vi "4.7.vi"() -> ()   [LabVIEW 2017]
panel:
  out "随机的数":i32
  out "猜了多少次":i32
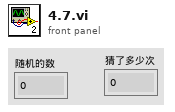
[diagram p1: front panel]
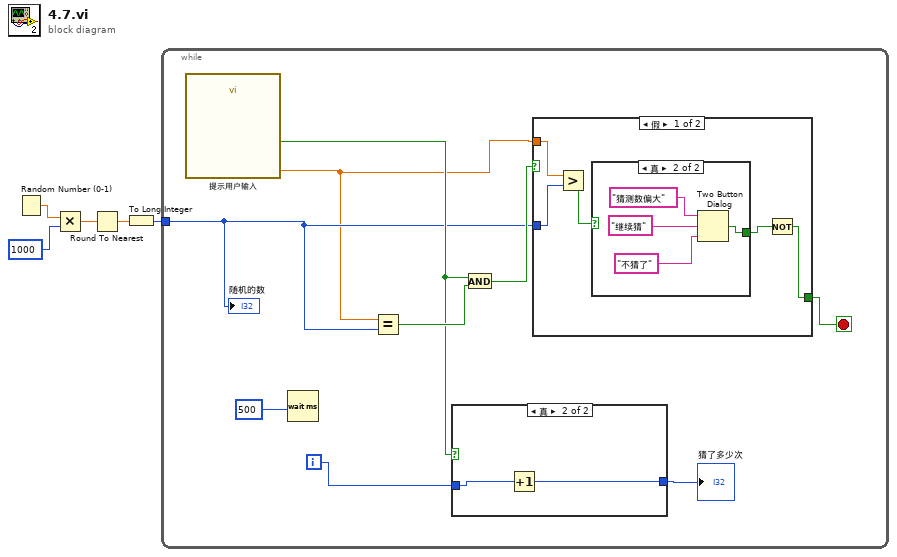
[diagram p0: block diagram]
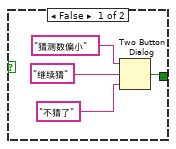
[diagram p3: hidden frame]
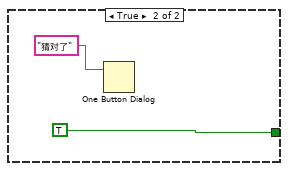
[diagram p4: hidden frame]
diagram:
  n1 = Random Number (0-1)() -> (number: 0 to 1=w5:dbl)
  n2 = Multiply(x=w5, y=1000) -> (x*y=w3:dbl)
  n3 = Round To Nearest(number=w3) -> (nearest integer value=w2:dbl)
  n4 = To Long Integer(number=w2) -> (32bit integer=w1:i32)
  n5 = while {
    tunnel: w1 -> [w9]
    i -> [w14]
    stop <- w7 stop-if-true
    n6 = call "提示用户输入"() -> ("请输入一个数"=w8:dbl, "确定"=w11:bool)  [unwired: 17 in, 1 out]
    n7 = Wait (ms)(milliseconds to wait=500) -> ()  [unwired: 1 out]
    n8 = Equal?(x=w8, y=w9) -> (x = y?=w12:bool)
    n9 = case shown="真" w11 {
      tunnel: w14 -> [_ w16]
      tunnel: [_ w15] -> w13
      frame False {
      }
      frame True {
        n10 = Increment(x=w16) -> (x+1=w15:i32)
      }
    }
    "猜了多少次" <- w13
    n11 = And(x=w11, y=w12) -> (x .and. y?=w10:bool)
    n12 = case shown="假" w10 {
      tunnel: w9 -> [w20 _]
      tunnel: w8 -> [w21 _]
      tunnel: [w17 TRUE] -> w7
      frame False {
        n13 = Greater?(x=w21, y=w20) -> (0:w19:bool)
        n14 = case shown="真" w19 {
          tunnel: [w23 w26] -> w18
          frame False {
            n15 = Two Button Dialog(message="猜测数偏小", 1:"不猜了", 2:"继续猜") -> (T button?=w23:bool)
          }
          frame True {
            n16 = Two Button Dialog(message="猜测数偏大", 1:"不猜了", 2:"继续猜") -> (T button?=w26:bool)
          }
        }
        n17 = Not(x=w18) -> (.not. x?=w17:bool)
      }
      frame True {
        n18 = One Button Dialog(message="猜对了") -> ()  [unwired: 1 in, 1 out]
      }
    }
    "随机的数" <- w9
  }
